vi "Get Trigger Mode.vi"(8 "error in (no error)":errorcluster, 11 "hdl":i32) -> (0 "error out":errorcluster, 2 "Trigger Mode":T1, 3 "hdl out":i32)   [LabVIEW 2013, in "Thorlabs_SC10.lvlib"]
uses:
  <instrlib>/Thorlabs_SC10/Thorlabs_SC10.lvlib
  <instrlib>/Thorlabs_SC10/Public/Configure/Trigger Mode.ctl
  <instrlib>/Thorlabs_SC10/Data/SC10CommandLib_x64.dll
  <instrlib>/Thorlabs_SC10/Data/SC10CommandLib_win32.dll
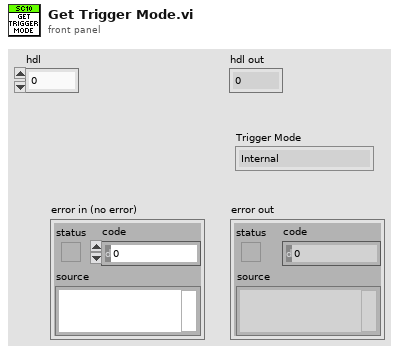
[diagram p1: front panel]
types:
  T1 = typedef "Thorlabs_SC10.lvlib/Trigger Mode.ctl" = enum16{"Internal", "External"}
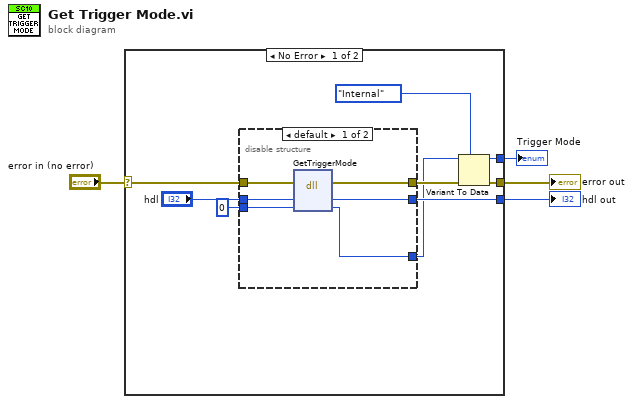
[diagram p0: block diagram]
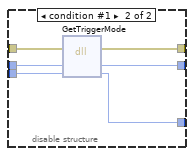
[diagram p2: hidden frame]
diagram:
  n1 = case shown="No Error" "error in (no error)" {
    selector: "error in (no error)" -> [w13 w26]
    tunnel: [w8 w26] -> w4
    tunnel: [w11 _] -> w2
    tunnel: [w5 _] -> w1
    frame No Error {
      n2 = disable-structure shown="default" {
        disable-tunnel: w13 -> [w19 w25]
        disable-tunnel: [w18 w24] -> w12
        disable-tunnel: [w17 w23] -> w11
        disable-tunnel: "hdl" -> [w16 w22]
        disable-tunnel: 0 ("value") -> [w15 w21]
        disable-tunnel: [w14 w20] -> w7
        frame condition #0 (active) {
          n3 = dll-call lib="C:/Program Files (x86)/National Instruments/LabVIEW 2013/instr.lib/Thorlabs_SC10/Data/SC10CommandLib_win32.dll" fn="GetTriggerMode"(error in=w19, "hdl"=w16, "value"=w15) -> (error out=w18:errorcluster, "hdl"=w17:i32, "value"=w14:i32)  [unwired: 3 in, 1 out]
        }
        frame condition #1 {
          n4 = dll-call lib="C:/Program Files/National Instruments/LabVIEW 2013/instr.lib/Thorlabs_SC10/Data/SC10CommandLib_x64.dll" fn="GetTriggerMode"(error in=w25, "hdl"=w22, "value"=w21) -> (error out=w24:errorcluster, "hdl"=w23:i32, "value"=w20:i32)  [unwired: 3 in, 1 out]
        }
      }
      n5 = Variant To Data(error in=w12, type=Trigger_Mode."Internal" ("Trigger Mode"), Variant=w7) -> (data=w5:T1, error out=w8:errorcluster)
    }
    frame Error {
    }
  }
  "error out" <- w4
  "hdl out" <- w2
  "Trigger Mode" <- w1
